vi "Main.vi"(8 "error in":errorcluster, 11 "File manipulate in":refnum<class "File manipulate.lvclass">) -> (0 "error out":errorcluster, 3 "File manipulate out":refnum<class "File manipulate.lvclass">)   [LabVIEW 2024, in "File manipulate.lvclass"]
doc: "The <b>Queued Message Handler</b> of the Worker that owns this VI."
uses:
  File manipulate.lvclass
  Initialization Data.ctl
  Response Cases.ctl
  File manipulate.lvclass/File manipulate.ctl
  rqp_Save Spectrogramme Data.ctl
  UI SmarAct/UI SmarAct.lvclass
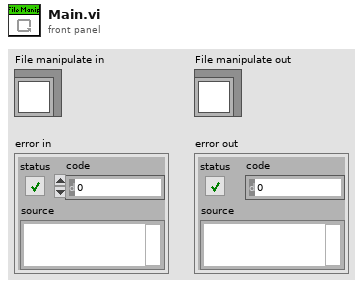
[diagram p1: front panel]
types:
  T1 = enum32{"Invalid", "Standard", "Closed", "Hidden", "Minimized", "Maximized"}
  T2 = typedef "File manipulate.lvclass/Initialization Data.ctl" = cluster{"Response Cases":T3}
  T3 = typedef "File manipulate.lvclass/Response Cases.ctl" = cluster{"Placeholder - Can be deleted":string}
  T4 = typedef "File manipulate.lvclass/rqp_Save Spectrogramme Data.ctl" = cluster{"Save SpecTG":bool, "Paramètres longueur d'onde":T5, "FROG Trace":dbl[][], "pas (um)":dbl, "Nbre de scans":i32, "WL Values":dbl[]}
  T5 = typedef "UI SmarAct.lvclass/Paramètres longueur d'onde.ctl" = cluster{"N":i32, "lambda_0":dbl, "lambda_c":dbl, "d_lambda":dbl}
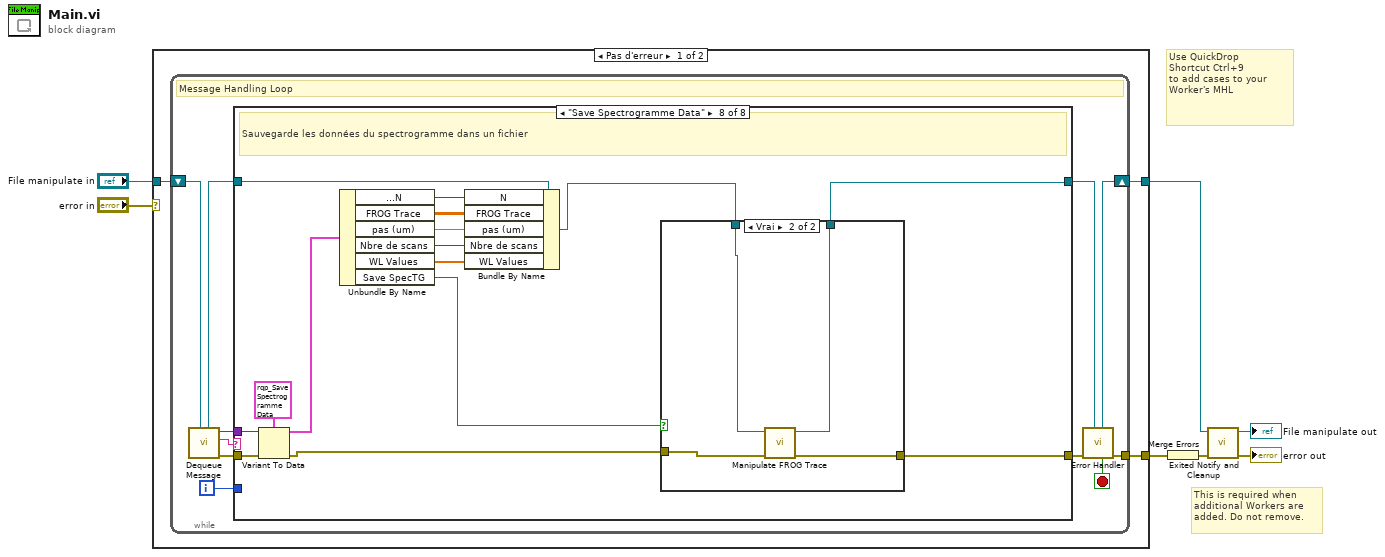
[diagram p0: block diagram]
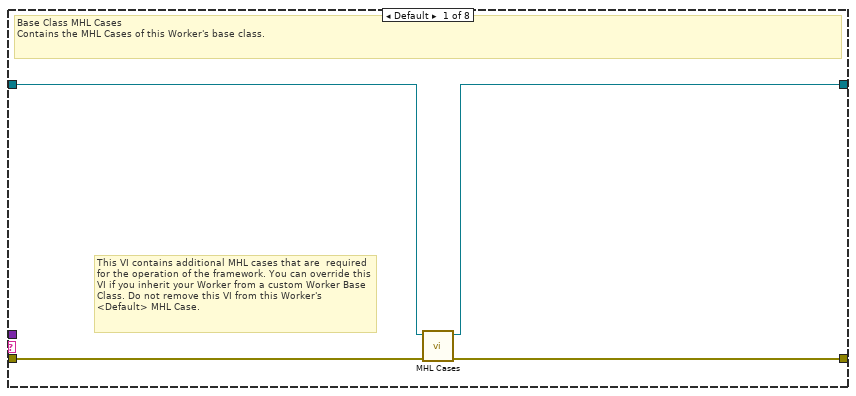
[diagram p2: hidden frame]
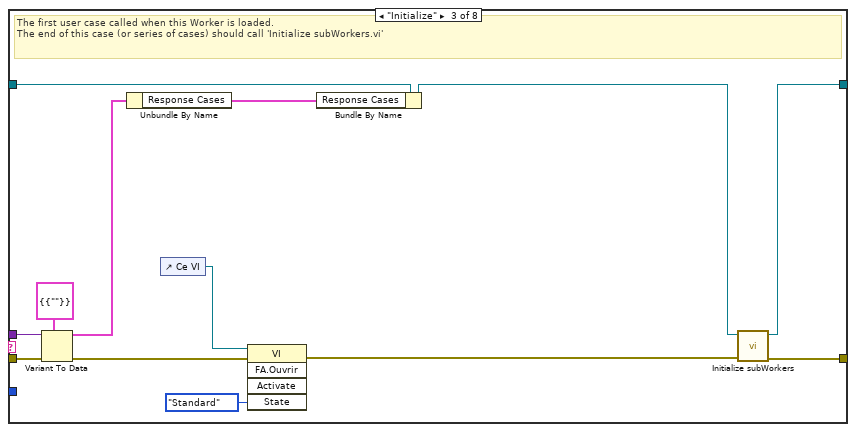
[diagram p4: hidden frame]
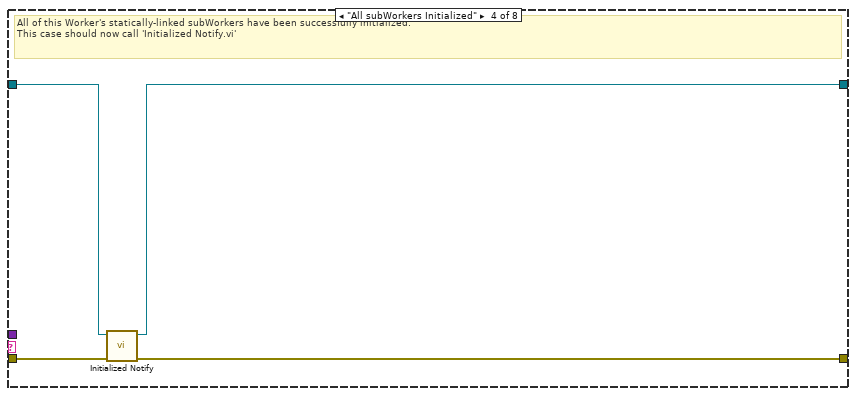
[diagram p5: hidden frame]
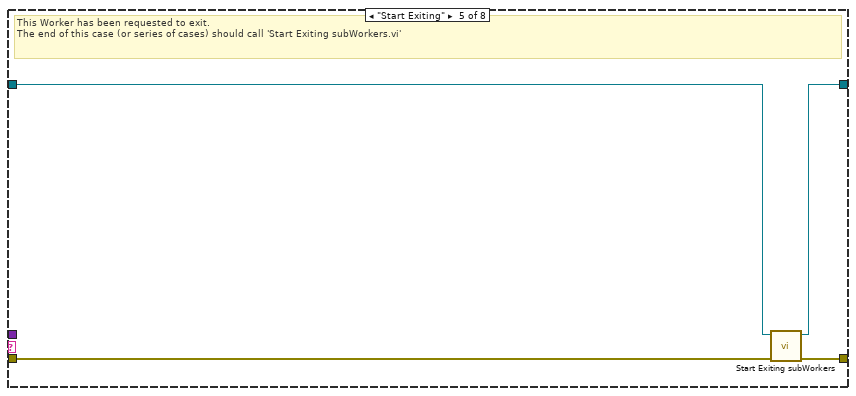
[diagram p6: hidden frame]
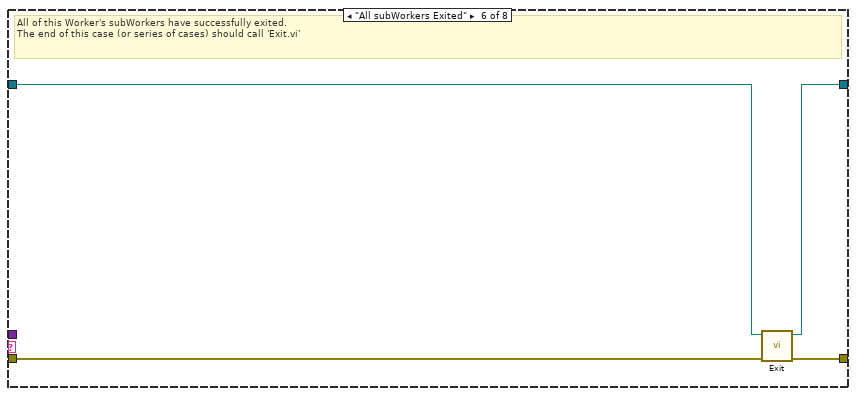
[diagram p7: hidden frame]
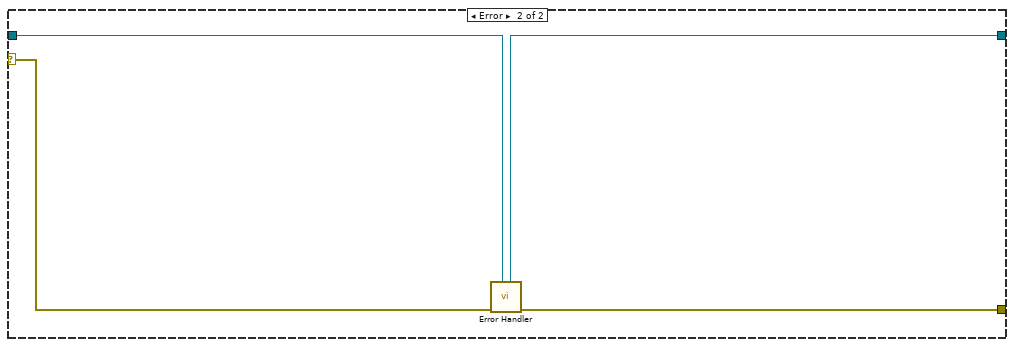
[diagram p10: hidden frame]
diagram:
  # "Use QuickDrop\nShortcut Ctrl+9\nto add cases to your\nWorker's MHL"
  # "This is required when additional Workers are added. Do not remove."
  n1 = case shown="Pas d'erreur" "error in" {
    tunnel: "File manipulate in" -> [w8 w77]
    tunnel: [w10 w78] -> w6
    tunnel: [w9 w76] -> w7
    selector: "error in" -> [_ w79]
    frame No Error {
      n2 = while {
        shift-right: [w19] -> w9
        shift-left: w8 -> [w21]
        tunnel: [w20] -> w10
        i -> [w12]
        stop <- w13 stop-if-true
        # "Message Handling Loop"
        n3 = call-dynamic "Dequeue Message.vi"("Worker"=w21) -> ("error out"=w18:errorcluster, "Case out"=w14:string, "Data out"=w11:variant, "Worker out"=w16:refnum<class "File manipulate.lvclass">)  [unwired: 6 in, 1 out]
        n4 = case "Worker MHL Case Structure (DO NOT CHANGE LABEL NAME)" shown="\"Save Spectrogramme Data\"" w14 {
          tunnel: w18 -> [w25 w26 w38 w44 w45 w52 w54 w69]
          tunnel: [w24 w26 w40 w43 w48 w51 w54 w65] -> w17
          tunnel: w16 -> [w23 w27 w37 w42 w46 w50 w53 w61]
          tunnel: [w22 w27 w39 w41 w47 w49 w53 w62] -> w15
          tunnel: w12 -> [_ _ _ _ _ _ _ _]
          tunnel: w11 -> [_ _ w36 _ _ _ _ w67]
          frame Default {
            # "This VI contains additional MHL cases that are  required for the operation of the framework. You can override this VI if you inherit your Worker from a custom Worker Base Class. Do not remove this VI from this Worker's <Default> MHL Case."
            # "Base Class MHL Cases\nContains the MHL Cases of this Worker's base class."
            n5 = call-dynamic "MHL Cases.vi"("error in"=w25, "Worker in"=w23) -> ("error out"=w24:errorcluster, "Worker out"=w22:refnum<class "File manipulate.lvclass">)  [unwired: 8 in]
          }
          frame "------------ FRAMEWORK CASES -----------" {
            # "Start of Workers Framework Cases"
          }
          frame "Initialize" {
            # "The first user case called when this Worker is loaded.\nThe end of this case (or series of cases) should call 'Initialize subWorkers.vi'"
            n6 = Variant To Data(error in=w38, type=T2 {"Response Cases"={"Placeholder - Can be deleted"=""}} ("Cluster"), Variant=w36) -> (data=w34:T2, error out=w31:errorcluster)
            n7 = Unbundle By Name(w34) -> ("Response Cases"=w33:T3)
            n8 = control-ref of="Ce VI"() -> (w30:refnum<vi>)
            n9 = invoke class="VI" method="FA.Ouvrir"(reference=w30, error in=w31, "State"=T1."Standard" ("État")) -> (error out=w29:errorcluster)  [unwired: 2 in, 4 out]
            n10 = Bundle By Name(cluster=w37, "Response Cases"=w33) -> (w35:refnum<class "File manipulate.lvclass">)
            n11 = call-dynamic "Initialize subWorkers.vi"("error in"=w29, "Worker"=w35) -> ("error out"=w40:errorcluster, "dup Worker out"=w39:refnum<class "File manipulate.lvclass">)  [unwired: 8 in]
          }
          frame "All subWorkers Initialized" {
            # "All of this Worker's statically-linked subWorkers have been successfully initialized.\nThis case should now call 'Initialized Notify.vi'"
            n12 = call-dynamic "Initialized Notify.vi"("error in"=w44, "Worker"=w42) -> ("error out"=w43:errorcluster, "dup Worker out"=w41:refnum<class "File manipulate.lvclass">)  [unwired: 8 in]
          }
          frame "Start Exiting" {
            # "This Worker has been requested to exit. \nThe end of this case (or series of cases) should call 'Start Exiting subWorkers.vi'"
            n13 = call-dynamic "Start Exiting subWorkers.vi"("error_in"=w45, "Worker"=w46) -> ("error out"=w48:errorcluster, "dup Worker out"=w47:refnum<class "File manipulate.lvclass">)  [unwired: 8 in]
          }
          frame "All subWorkers Exited" {
            # "All of this Worker's subWorkers have successfully exited. \nThe end of this case (or series of cases) should call 'Exit.vi'"
            n14 = call-dynamic "Exit.vi"("error_in"=w52, "Worker"=w50) -> ("error out"=w51:errorcluster, "dup Worker out"=w49:refnum<class "File manipulate.lvclass">)  [unwired: 8 in]
          }
          frame "------------- PUBLIC API CASES -------------" {
            # "Start of Workers Public API Cases"
          }
          frame "Save Spectrogramme Data" {
            # "Sauvegarde les données du spectrogramme dans un fichier"
            n15 = Variant To Data(error in=w69, type=T4 {"Save SpecTG"=FALSE, "Paramètres longueur d'onde"={"N"=2068, "lambda_0"=200.6310762, "lambda_c"=674.8888701568728, "d_lambda"=0.44435503366880597}, "FROG Trace"=[], "pas (um)"=0.0, "Nbre de scans"=0, "WL Values"=[]} ("Data"), Variant=w67) -> (data=w66:T4, error out=w64:errorcluster)
            n16 = Unbundle By Name(w66) -> ("Paramètres longueur d'onde.N"=w59:i32, "FROG Trace"=w58:dbl[][], "pas (um)"=w57:dbl, "Nbre de scans"=w56:i32, "WL Values"=w55:dbl[], "Save SpecTG"=w63:bool)
            n17 = Bundle By Name(cluster=w61, "N"=w59, "FROG Trace"=w58, "pas (um)"=w57, "Nbre de scans"=w56, "WL Values"=w55) -> (w60:refnum<class "File manipulate.lvclass">)
            n18 = case shown="Vrai" w63 {
              tunnel: [w71 w74] -> w65
              tunnel: w64 -> [w71 w75]
              tunnel: [w70 w72] -> w62
              tunnel: w60 -> [w70 w73]
              frame False {
              }
              frame True {
                n19 = call "Manipulate FROG Trace.vi"("error in (no error)"=w75, "File mainpulate en entrée"=w73) -> ("error out"=w74:errorcluster, "File mainpulate en sortie"=w72:refnum<class "File manipulate.lvclass">)  [unwired: 8 in]
              }
            }
          }
        }
        n20 = call-dynamic "Error Handler.vi"("Worker"=w15, "error_in"=w17) -> ("error out"=w20:errorcluster, "Stop Loop"=w13:bool, "Worker out"=w19:refnum<class "File manipulate.lvclass">)  [unwired: 7 in]
      }
    }
    frame Error {
      n21 = call-dynamic "Error Handler.vi"("Worker"=w77, "error_in"=w79) -> ("error out"=w78:errorcluster, "Worker out"=w76:refnum<class "File manipulate.lvclass">)  [unwired: 7 in, 1 out]
    }
  }
  n22 = Merge Errors(w6) -> (w3:errorcluster)
  n23 = call-dynamic "Exited Notify and Cleanup.vi"("error_in"=w3, "Worker"=w7) -> ("error out"=→"error out":errorcluster, "dup Worker out"=→"File manipulate out":refnum<class "File manipulate.lvclass">)  [unwired: 8 in]
